vi "Set Charge Shifting.vi"(10 "NumberRepeats":u32, 11 "NumberRows":u32) -> (3 "function return":u32)   [LabVIEW 2018, in "AndorSDK.lvlib"]
doc: "EXPNETTYPE unsigned int WINAPI SetChargeShifting(unsigned int NumberRows, unsigned int NumberRepeats);"
uses:
  AndorSDK.lvlib
  ATMCD32D.dll
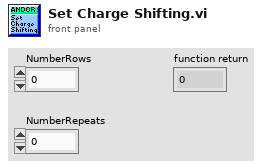
[diagram p1: front panel]
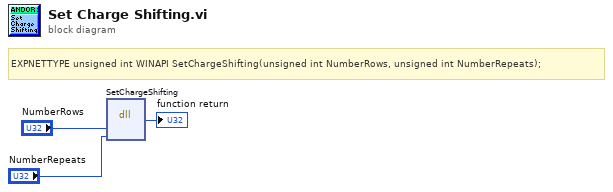
[diagram p0: block diagram]
diagram:
  # "EXPNETTYPE unsigned int WINAPI SetChargeShifting(unsigned int NumberRows, unsigned int NumberRepeats);"
  n1 = dll-call lib="PTH2babs E\nPersönliches02 - Arbeit03-HiwijobsLabviewCodelibANDOR\tAndor SDK\nATMCD32D.*" fn="SetChargeShifting"("NumberRows"="NumberRows", "NumberRepeats"="NumberRepeats") -> (→"function return":u32)  [unwired: 5 in, 2 out]
